vi "FTW-JSON-ObjectManip-Update.vi"(0 "Input JSON Object":string, 5 "JSON Object to Merge":string, 7 "Update Mode":T1, 11 "error in":errorcluster) -> (4 "Output JSON Object":string, 15 "error out":errorcluster)   [LabVIEW 2015]
uses:
  FTW-JSON-JoinMode.ctl
panel:
  # "Inputs"
  # "Outputs"
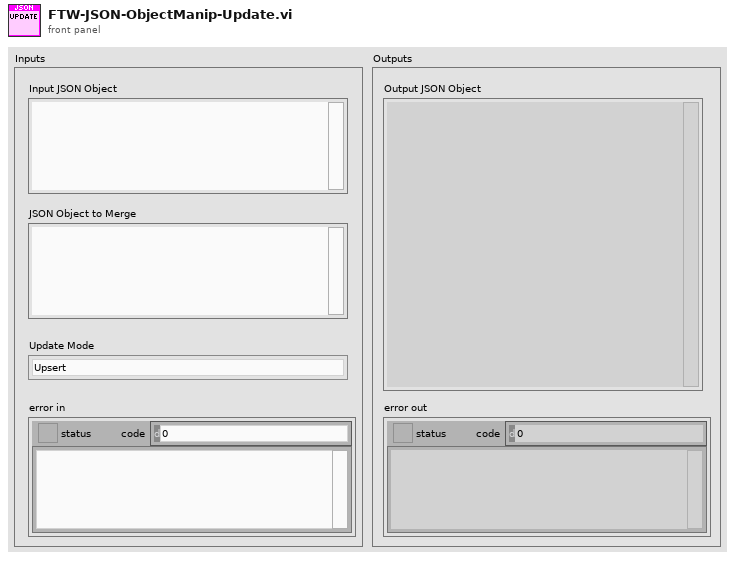
[diagram p1: front panel]
types:
  T1 = typedef "FTW-JSON-JoinMode.ctl" = enum32{"Upsert", "Update Only", "Insert Only"}
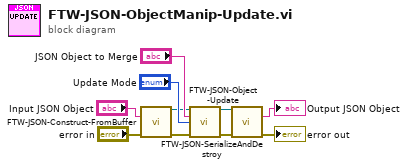
[diagram p0: block diagram]
diagram:
  n1 = call "FTW-JSON-Construct-FromBuffer.vi"("JSON String (UTF-8)"="Input JSON Object", "error in"="error in") -> ("JSON"=w3:refnum<class "FTW-Container.lvclass">, "error out"=w5:errorcluster)  [unwired: 12 in]
  n2 = call "FTW-JSON-Object-Update.vi"("JSON Object"=w3, "JSON Object to Merge"="JSON Object to Merge", "Update Mode"="Update Mode", "error in"=w5) -> ("JSON Object out"=w2:refnum<class "FTW-Container.lvclass">, "error out"=w4:errorcluster)  [unwired: 10 in]
  n3 = call "FTW-JSON-SerializeAndDestroy.vi"("JSON"=w2, "error in"=w4) -> ("JSON String (UTF-8)"=→"Output JSON Object":string, "error out"=→"error out":errorcluster)  [unwired: 12 in]
